vi "TCP Connection Manager.vi"(6 "Properties In":T1, 8 "error in (no error)":errorcluster, 9 "Method":T4, 10 "Index":i32, 11 "Connection In":T2) -> (0 "error out":errorcluster, 1 "Number of Connections":i32, 2 "All Connections":T2[](array[typedef]), 3 "Connection Out":T2, 4 "Properties out":T1, 5 "All Properties":T1[](array[typedef]))   [LabVIEW 2010]
doc: "This VI maintains the list of host connections."
uses:
  stm_TCPConnectionMethod.ctl
  stm_TCP Connection Info.ctl
  stm_MetaDataElement.ctl
  stm_TCPConnectionProperties.ctl
  NI STM.lvlib
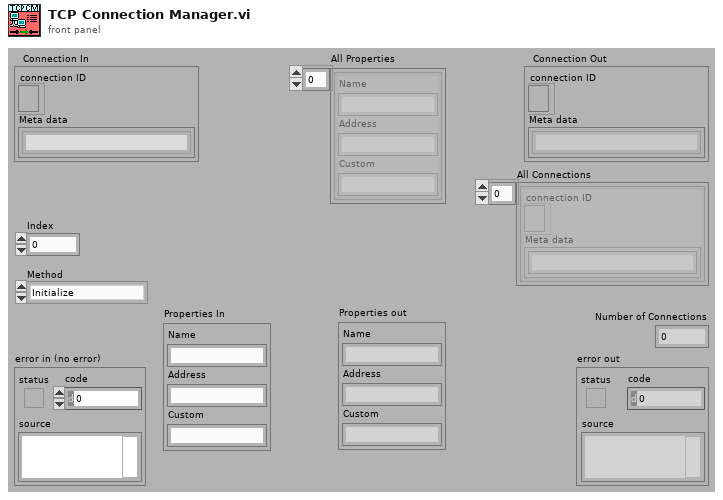
[diagram p1: front panel]
types:
  T1 = typedef "stm_TCPConnectionProperties.ctl" = cluster{"Name":string, "Address":string, "Custom":string}
  T2 = typedef "stm_TCP Connection Info.ctl" = cluster{"connection ID":refnum<k5>, "Meta data":T3[]}
  T3 = typedef "stm_MetaDataElement.ctl" = string
  T4 = typedef "stm_TCPConnectionMethod.ctl" = enum16{"Initialize", "Add Connection", "Set Properties", "Get Connection(s)", "Remove Connection", "Remove All Connections", "Get Connection Count"}
  T5 = typedef "NI STM.lvlib/TCP Connection Info.ctl" = cluster{"connection ID":refnum<k5>, "Meta data":T6[]}
  T6 = typedef "NI STM.lvlib/MetaDataElement.ctl" = string
  T7 = typedef "NI STM.lvlib/TCP Connection Properties.ctl" = cluster{"Name":string, "Address":string, "Custom":string}
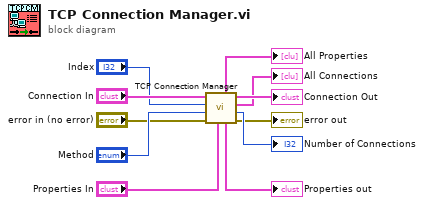
[diagram p0: block diagram]
diagram:
  n1 = call "TCP Connection Manager.vi"("Properties In"="Properties In", "error in"="error in (no error)", "Method"="Method", "Index"="Index", "Connection In"="Connection In") -> ("error out"=→"error out":errorcluster, "Number of Connections"=→"Number of Connections":i32, "All Connections"=→"All Connections":T5[], "Connection Out"=→"Connection Out":T5, "Properties out"=→"Properties out":T7, "All Properties"=→"All Properties":T7[])  [unwired: 1 in]
